vi "Color Decoration.vi"(0 "VI reference":refnum<vi>, 1 "Color Array":u32[](array[colorbox]), 2 "Index Array":u32[](array[numeric]), 3 "error in (no error)":errorcluster) -> (10 "error out":errorcluster)   [LabVIEW 2013]
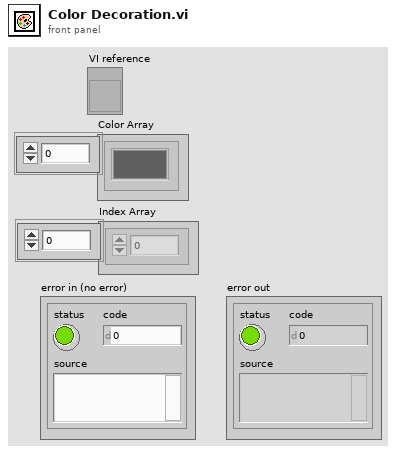
[diagram p1: front panel]
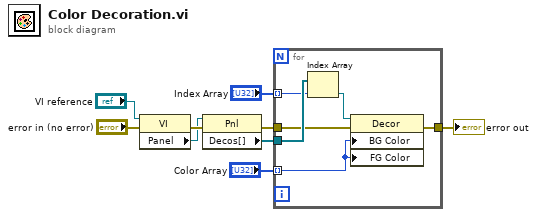
[diagram p0: block diagram]
diagram:
  n1 = property class="VI"(reference="VI reference", error in="error in (no error)") -> (error out=w9:errorcluster, "Panel"=w8:refnum<vi>)  [unwired: 1 out]
  n2 = property class="Pnl"(reference=w8, error in=w9) -> (error out=w1:errorcluster, "Decos[]"=w4:refnum<vi>[])  [unwired: 1 out]
  n3 = for {
    tunnel: "Index Array" -> [w14] mode=indexing
    tunnel: w4 -> [w15]
    tunnel: "Color Array" -> [w12] mode=indexing
    tunnel: [w11] -> w2
    tunnel: w1 -> [w10]
    n4 = Index Array(array=w15, index=w14) -> (element=w13:refnum<vi>)
    n5 = property class="Decor"(reference=w13, error in=w10, "BG Color"=w12, "FG Color"=w12) -> (error out=w11:errorcluster)  [unwired: 1 out]
  }
  "error out" <- w2
